vi "R I Monitorn Test Interface.vi"() -> ()   [LabVIEW 2012, in "Signal Analysis.lvlib"]
uses:
  Signal Analysis.lvlib
  <vilib>/Platform/TimedLoop/XDataNode/timing_clust.ctl
  <vilib>/Platform/TimedLoop/XDataNode/nitl_modes.ctl
  <vilib>/Platform/TimedLoop/XDataNode/wakeup.ctl
  <vilib>/Platform/TimedLoop/XDataNode/XDataNode.xnode
  <vilib>/measure/NI_MABase.lvlib
  <vilib>/Platform/TimedLoop/XDataNode/XDNodeRunTimeDep.lvlib
panel:
  in  "Multiclamp Reference":i32
  in  "Noise":dbl(knob) scale=0.0001..1000.0
  in  "Amplitude":dbl(knob) scale=0.0001..1000.0
  in  "Filter":T1={"Topology"=enum."Bessel", "Type"=enum."Lowpass", "Order"=1, "Lower Fc"=3000.0, "Upper Fc"=200.0, "PB Ripple"=1.0, "SB Attenuation"=60.0}
  out "Resistance":dbl(graph)
  out "Current":dbl(graph)
  in  "Filter On":bool=TRUE
  in  "On/Off":bool=TRUE
  out "Waveform Graph":waveform(dbl)(graph)
  in  "stop":bool
  in  "error in (no error)":errorcluster
  out "error out":errorcluster
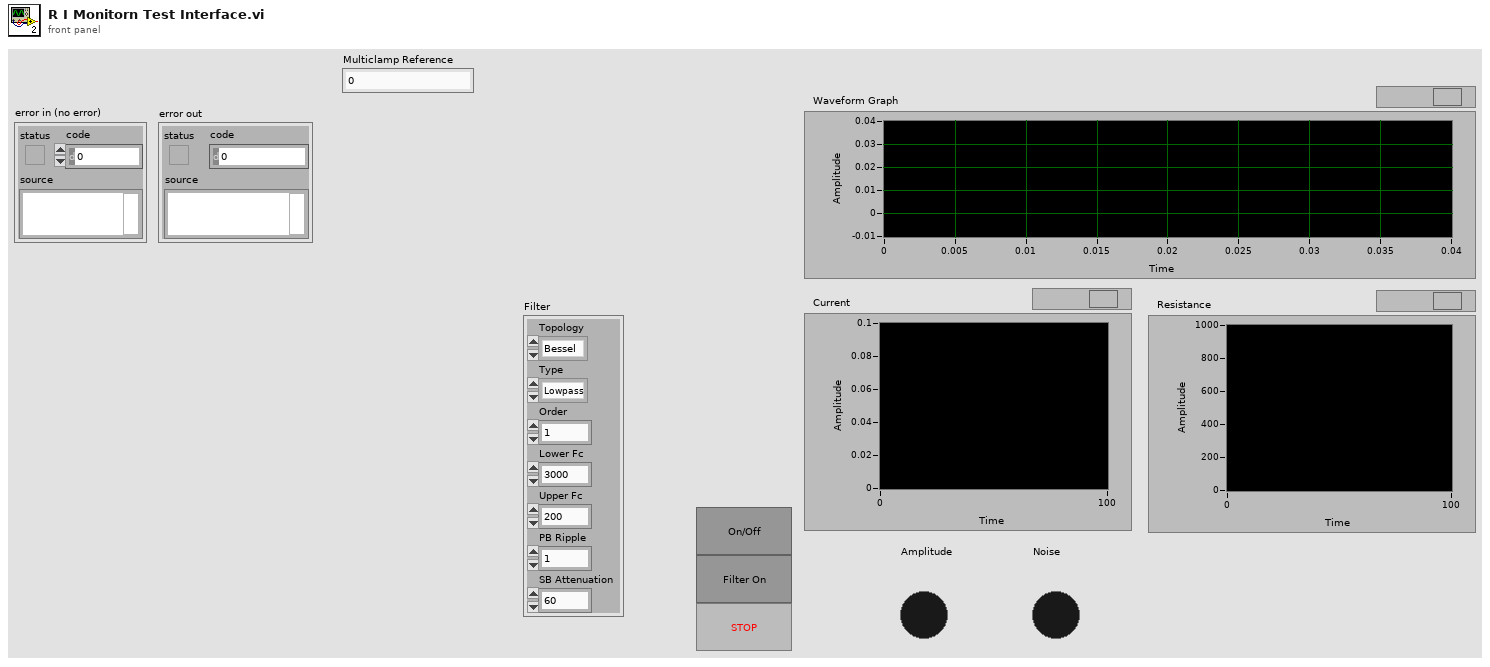
[diagram p1: front panel]
types:
  T1 = cluster{"Topology":enum16{"Off", "Butterworth", "Chebyshev", "Inverse Chebyshev", "Elliptic", "Bessel"}, "Type":enum16{"Lowpass", "Highpass", "Bandpass", "Bandstop"}, "Order":i32, "Lower Fc":dbl, "Upper Fc":dbl, "PB Ripple":dbl, "SB Attenuation":dbl}
  T2 = cluster{"On/Off":refnum<vi>, "Filter On/Off":refnum<vi>, "Stop":refnum<vi>, "IIR filter specifications":refnum<vi>}
  T3 = typedef "XDNodeRunTimeDep.lvlib/timing_clust.ctl" = cluster{"Expected End [f-1]":u64, "Actual End [f-1]":u64, "Finished Late? [f-1]":bool, "Expected End [i-1]":u64, "Actual End [i-1]":u64, "Finished Late? [i-1]":bool, "Expected Start [i]":u64, "Actual Start [i]":u64, "Expected Start [f]":u64, "Actual Start [f]":u64, "Source Name":string, "Structure Name":string, "Period":i64, "Deadline":i64, "Offset":i64, "Start":i64, "Priority":i32, "Timeout":i32, "Mode":T4, "Wakeup Reason":T5, "Error":errorcluster, "Source Type":string, "Secondary Source Type":string, "Global End Time":u64, "Global Start Time":u64, "Frame Duration":u64, "Iteration Duration":u64, "Assigned CPU":i32, "I/O Scan Engine Mode":u32}
  T4 = typedef "XDNodeRunTimeDep.lvlib/nitl_modes.ctl" = enum32{"No Change", "Process missed periods, maintain original phase", "Discard missed periods, maintain original phase", "Process missed periods, ignore original phase", "Discard missed periods, ignore original phase"}
  T5 = typedef "XDNodeRunTimeDep.lvlib/wakeup.ctl" = enum32{"Normal", "Aborted", "Asynchronous wakeup", "Timing source error", "Timed loop error", "Timeout"}
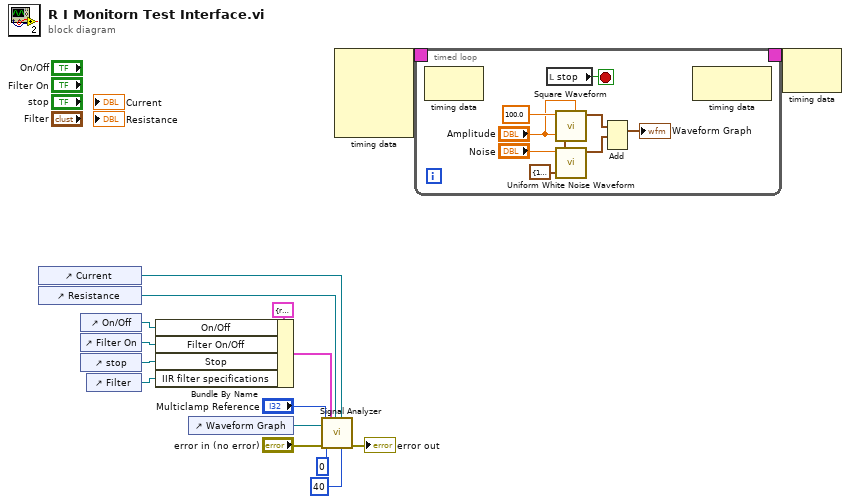
[diagram p0: block diagram]
diagram:
  n1 = control-ref of="Current"() -> (w1:refnum<vi>)
  n2 = control-ref of="Resistance"() -> (w2:refnum<vi>)
  n3 = control-ref of="On/Off"() -> (w12:refnum<vi>)
  n4 = control-ref of="Filter On"() -> (w11:refnum<vi>)
  n5 = control-ref of="stop"() -> (w13:refnum<vi>)
  n6 = control-ref of="Filter"() -> (w10:refnum<vi>)
  n7 = Bundle By Name(cluster=T2 {"On/Off"=refnum, "Filter On/Off"=refnum, "Stop"=refnum, "IIR filter specifications"=refnum} ("Controllers"), "On/Off"=w12, "Filter On/Off"=w11, "Stop"=w13, "IIR filter specifications"=w10) -> (w3:T2)
  n8 = control-ref of="Waveform Graph"() -> (w14:refnum<vi>)
  n9 = call "Signal Analyzer.vi"("Period [ms]"=i64 40, "Current"=w1, "Controllers"=w3, "Resistance"=w2, "error in (no error)"="error in (no error)", "Multiclamp Error"=0, "Multiclamp Reference"="Multiclamp Reference", "Test Signal"=w14) -> ("error out"=→"error out":errorcluster)  [unwired: 1 in, 2 out]
  n10 = node-c288() -> (w9:T3)  [unwired: 4 in]
  n11 = timed-loop {
    timing: w9 -> [_]
    timing-out: [_] -> w8
    stop <- w19 stop-if-true
    w20 = cluster{"Fs":dbl, "#s":dbl} {"Fs"=10000.0, "#s"=10000.0} ("sampling info")
    n12 = node-c288() -> ()  [unwired: 1 in, 1 out]
    n13 = local read "stop"() -> (w19:bool)
    n14 = call <vilib>:"Square Waveform.vi"("offset"="Amplitude", "sampling info"=w20, "amplitude"="Amplitude", "frequency"=100.0) -> ("signal out"=w23:waveform(dbl))  [unwired: 6 in, 1 out]
    n15 = call <vilib>:"Uniform White Noise Waveform.vi"("sampling info"=w20, "amplitude"="Noise") -> ("signal out"=w22:waveform(dbl))  [unwired: 8 in, 1 out]
    n16 = Add(1:w22, 2:w23) -> (0:→"Waveform Graph":waveform(dbl))  [unwired: 1 in, 1 out]
    n17 = node-c288() -> ()  [unwired: 1 in, 1 out]
  }
  n18 = node-c288(w8) -> ()  [unwired: 1 out]
